vi "FindEyes_LVPic.vi"(8 "error in (no error)":errorcluster, 10 "2D Picture in":picture, 11 "reference in":refnum<class "ImageFacialDetection.lvclass">) -> (0 "error out":errorcluster, 2 "2D Picture out":picture, 3 "reference out":refnum<class "ImageFacialDetection.lvclass">)   [LabVIEW 2017, in "ImageFacialDetection.lvclass"]
doc: "finds faces on an IMAQ image"
uses:
  ImageFacialDetection.lvclass
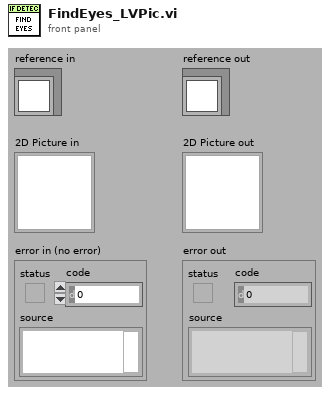
[diagram p1: front panel]
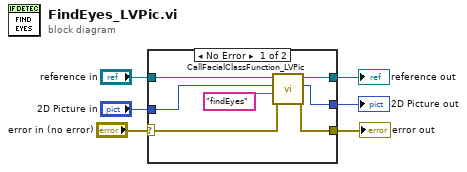
[diagram p0: block diagram]
diagram:
  n1 = case shown="No Error" "error in (no error)" {
    selector: "error in (no error)" -> [w9 w15]
    tunnel: [w8 w15] -> w5
    tunnel: [w12 w14] -> w3
    tunnel: "reference in" -> [w13 w14]
    tunnel: "2D Picture in" -> [w11 _]
    tunnel: [w7 _] -> w1
    frame No Error {
      n2 = call "CallFacialClassFunction_LVPic.vi"("error in (no error)"=w9, "Function or Method Name"="findEyes", "image"=w11, "reference in"=w13) -> ("error out"=w8:errorcluster, "image with faces"=w7:picture, "reference out"=w12:refnum<class "ImageFacialDetection.lvclass">)  [unwired: 5 in]
    }
    frame Error {
    }
  }
  "error out" <- w5
  "reference out" <- w3
  "2D Picture out" <- w1
